vi "Binding Path to SHV.vi"() -> ()   [LabVIEW 2015]
panel:
  out "Colors [4]":cluster{u32, u32}[](array[cluster])
  in  "Sample 3":bool
  in  "shared variable":refnum<k21>
  out "String":string
  out "Numeric":i32
  out "Array":string[](array[string])
  out "path":path
  out "string":string
  in  "shared variable refnum in":refnum<k21>
  in  "Data Binding:Path":string="\\\\EGP-GAS\\AMS Gas SHV PC\\Sample Lines\\Line 1\\Sample In"
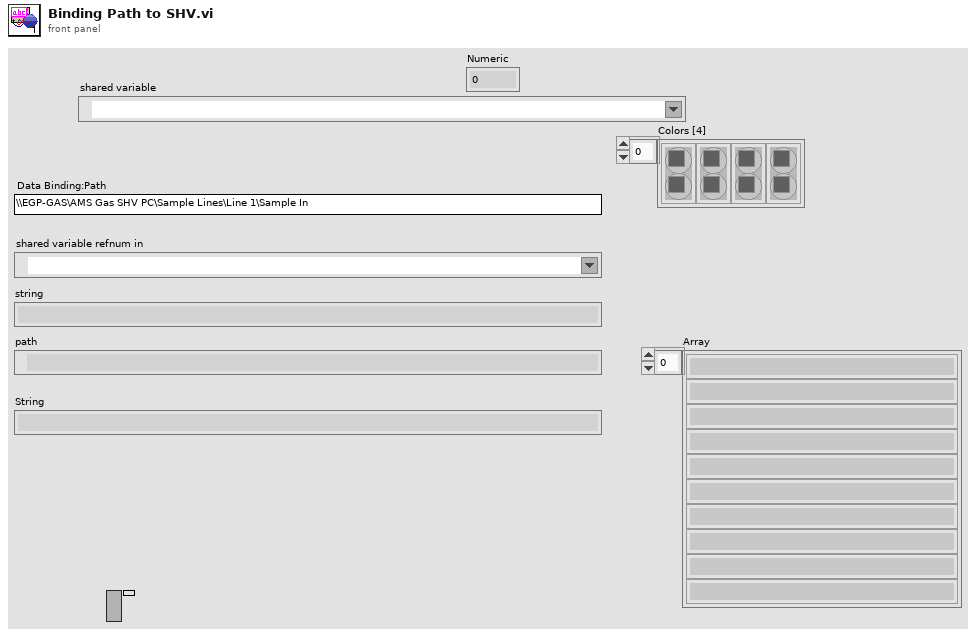
[diagram p1: front panel]
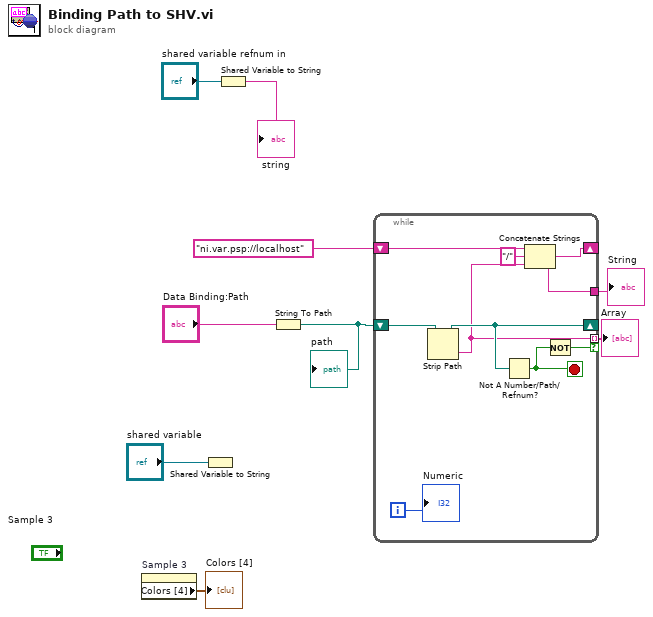
[diagram p0: block diagram]
diagram:
  n1 = property on="Sample 3" class="Bool (strict)"() -> ("Colors [4]"=→"Colors [4]":cluster{u32, u32}[])  [unwired: 2 in, 2 out]
  n2 = Shared Variable to String(1:"shared variable") -> ()  [unwired: 1 out]
  n3 = Shared Variable to String(1:"shared variable refnum in") -> (0:→"string":string)
  n4 = String To Path(string="Data Binding:Path") -> (path=w5:path)
  "path" <- w5
  n5 = while {
    shift-right: [w18] -> _
    shift-left: w5 -> [w16]
    tunnel: [w11] -> w7 mode=indexing if=w14
    shift-right: [w10] -> _
    shift-left: "ni.var.psp://localhost" -> [w13]
    tunnel: [w10] -> w3
    i -> [w15]
    stop <- w17 stop-if-true
    n6 = Strip Path(path=w16) -> (stripped path=w18:path, name=w11:string)
    n7 = Not A Number/Path/Refnum?(number/path/refnum=w18) -> (NaN/Path/Refnum?=w17:bool)
    n8 = Concatenate Strings(w13, "/" ("string"), w11) -> (w10:string)
    n9 = Not(x=w17) -> (.not. x?=w14:bool)
    "Numeric" <- w15
  }
  "Array" <- w7
  "String" <- w3
